vi "SeCrTs - RD obtain Queue.vi"(8 "error in":errorcluster) -> (0 "error out":errorcluster, 2 "Analog Queue":refnum<queue>[](array[refnum]), 3 "DI Data Queue":refnum<queue>)   [LabVIEW 2022 SP3]
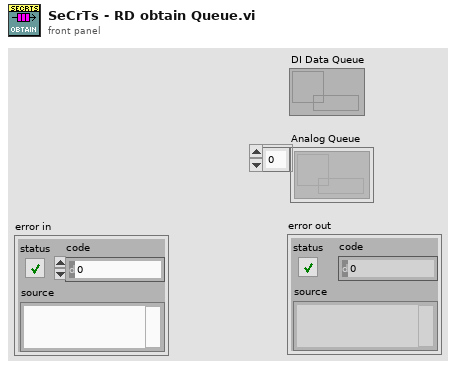
[diagram p1: front panel]
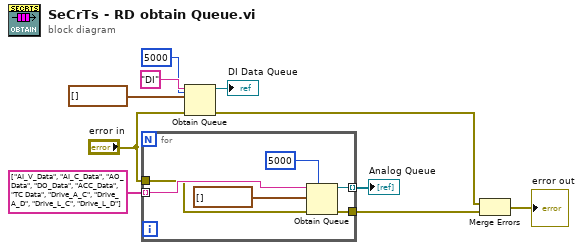
[diagram p0: block diagram]
diagram:
  n1 = for {
    tunnel: string[] ["AI_V_Data", "AI_C_Data", "AO_Data", "DO_Data", "ACC_Data", "TC Data", "Drive_A_C", "Drive_A_D", "Drive_L_C", "Drive_L_D"] ("Array") -> [w16] mode=indexing
    tunnel: "error in" -> [w14]
    tunnel: [w13] -> w4 mode=indexing
    tunnel: [w12] -> w3
    n2 = Obtain Queue(max queue size (-1, unlimited)=5000, name (unnamed)=w16, element data type=waveform(dbl)[] [] ("AI_V_Data"), error in (no error)=w14) -> (queue out=w13:refnum<queue>, error out=w12:errorcluster)  [unwired: 1 in, 1 out]
  }
  "Analog Queue" <- w4
  n3 = Obtain Queue(max queue size (-1, unlimited)=5000, name (unnamed)="DI", element data type=digitalwaveform[] [] ("DI_Data"), error in (no error)="error in") -> (queue out=→"DI Data Queue":refnum<queue>, error out=w1:errorcluster)  [unwired: 1 in, 1 out]
  n4 = Merge Errors(w1, w3) -> (→"error out":errorcluster)
